vi "password2.vi"(11 "error in (no error)":errorcluster) -> (4 "result":bool, 8 "This VI":refnum<vi>, 15 "error out":errorcluster)   [LabVIEW 2019]
panel:
  in  "Password":string
  in  "User Name":string
  out "String":string="Please insert User Name and Password"
  in  "Cancel":bool
  in  "OK2":bool
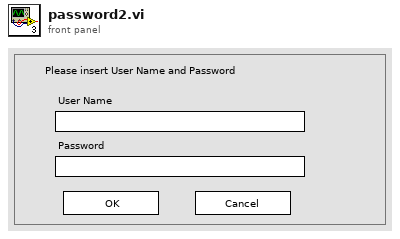
[diagram p1: front panel]
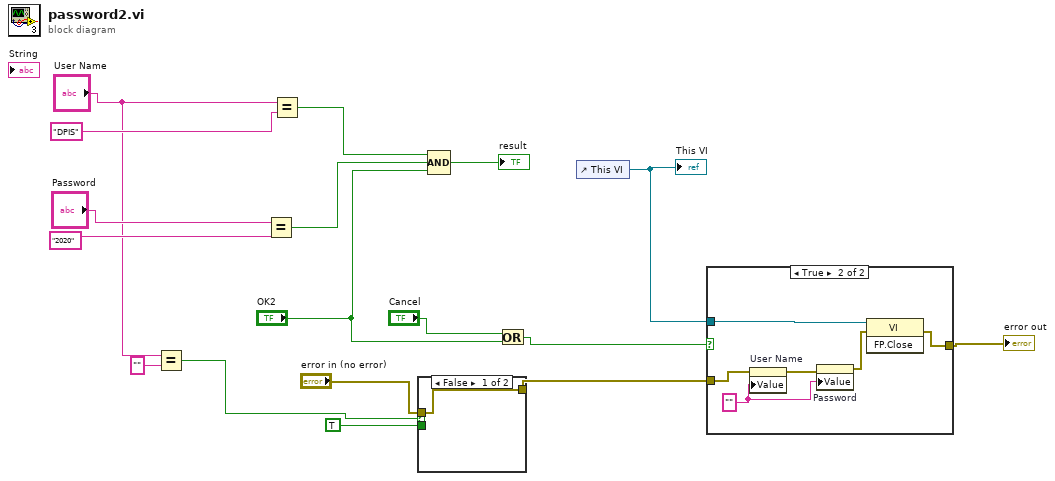
[diagram p0: block diagram]
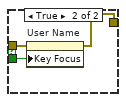
[diagram p2: hidden frame]
diagram:
  n1 = Equal?(x="User Name", y="") -> (x = y?=w1:bool)
  n2 = Equal?(x="Password", y="2020") -> (x = y?=w13:bool)
  n3 = Equal?(x="User Name", y="DPIS") -> (x = y?=w14:bool)
  n4 = case shown="False" w1 {
    tunnel: "error in (no error)" -> [w18 w21]
    tunnel: [w18 w20] -> w5
    tunnel: TRUE ("Key Focus") -> [_ w19]
    frame False {
    }
    frame True {
      n5 = property on="User Name" class="Str"(error in=w21, "Key Focus"=w19) -> (error out=w20:errorcluster)  [unwired: 1 in, 1 out]
    }
  }
  n6 = Compound Arithmetic op=AND(w14, w13, "OK2") -> (→"result":bool)
  n7 = Or(x="Cancel", y="OK2") -> (x .or. y?=w10:bool)
  n8 = control-ref of="This VI"() -> (w8:refnum<vi>)
  "This VI" <- w8
  n9 = case shown="True" w10 {
    tunnel: w8 -> [_ w28]
    tunnel: w5 -> [w22 w26]
    tunnel: [w22 w27] -> w7
    frame False {
    }
    frame True {
      w23 = "" ("User Name")
      n10 = property on="User Name" class="Str"(error in=w26, "Value"=w23) -> (error out=w25:errorcluster)  [unwired: 1 in, 1 out]
      n11 = property on="Password" class="Str"(error in=w25, "Value"=w23) -> (error out=w24:errorcluster)  [unwired: 1 in, 1 out]
      n12 = invoke class="VI" method="FP.Close"(reference=w28, error in=w24) -> (error out=w27:errorcluster)  [unwired: 1 in, 2 out]
    }
  }
  "error out" <- w7
